vi "Hardware Device Get All Info.vi"(8 "error in":errorcluster, 9 "Terminals":tag[](array[tag]), 11 "NI PWM Output in":refnum<class "NI PWM Output.lvclass">) -> (0 "error out":errorcluster, 1 "CO.PhysicalChans":tag[](array[tag]), 3 "NI PWM Output out":refnum<class "NI PWM Output.lvclass">)   [LabVIEW 2023, in "HardwareAbstractionLayer_LVOOP.lvlib" / "NI PWM Output.lvclass"]
doc: "This VI Device Physical Channel Read"
uses:
  NI PWM Output.lvclass
  NI PWM Output.lvclass/NI PWM Output.ctl
  <resource>/objmgr/daqmx.rc
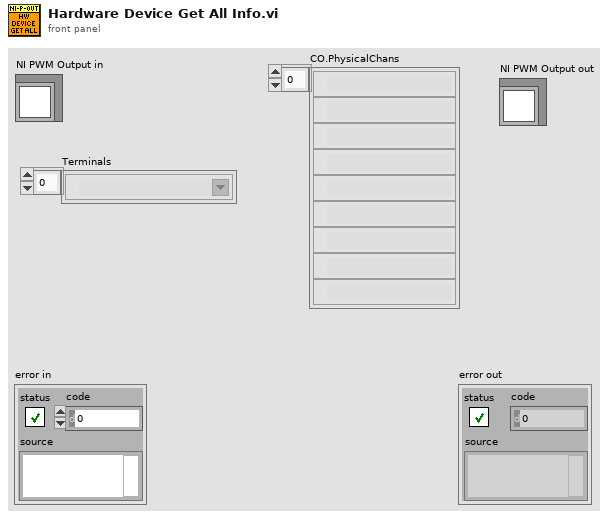
[diagram p1: front panel]
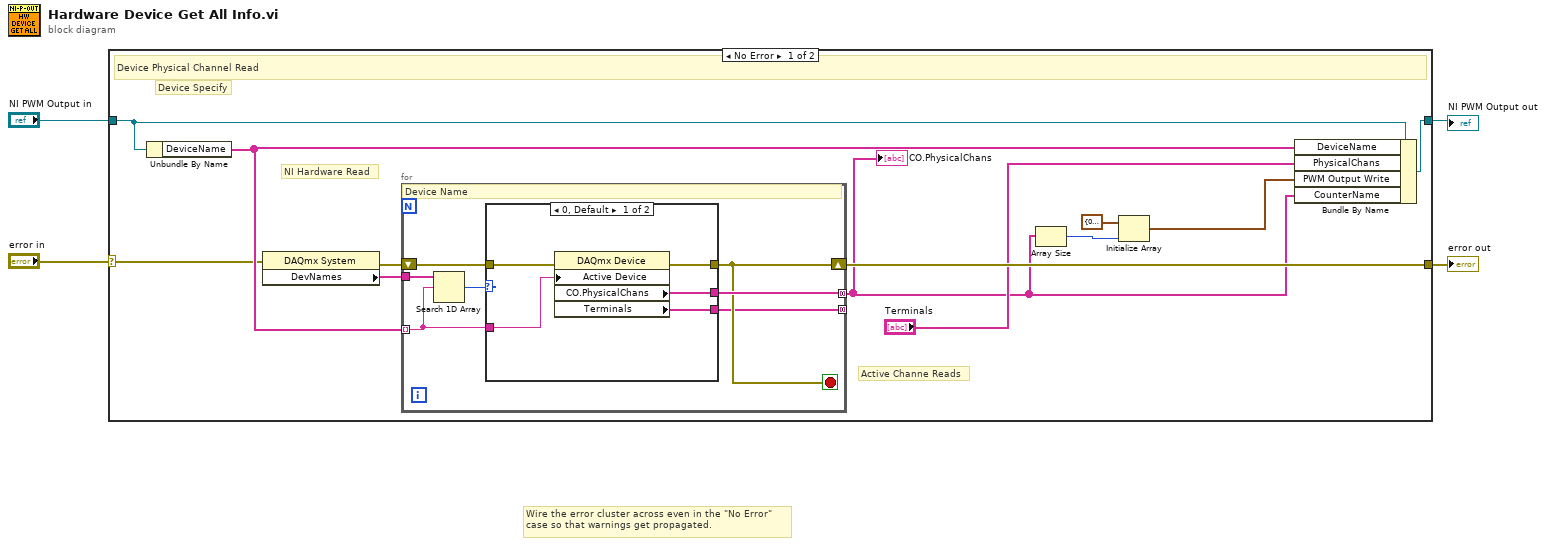
[diagram p0: block diagram]
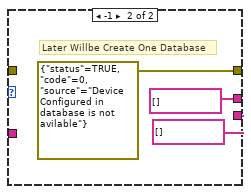
[diagram p2: hidden frame]
diagram:
  # "Wire the error cluster across even in the \"No Error\"\ncase so that warnings get propagated."
  n1 = case shown="No Error" "error in" {
    selector: "error in" -> [w7 w33]
    tunnel: [w8 w33] -> w3
    tunnel: [w13 w32] -> w1
    tunnel: "NI PWM Output in" -> [w12 w32]
    frame No Error {
      # "Active Channe Reads"
      # "Device Specify"
      # "NI Hardware Read"
      # "Device Physical Channel Read"
      n2 = Unbundle By Name(w12) -> ("DeviceName"=w16:tag[])
      n3 = property class="DAQmx System"(error in=w7) -> (error out=w14:errorcluster, "DevNames"=w15:tag[])  [unwired: 1 in, 1 out]
      n4 = for {
        tunnel: w16 -> [w20] mode=indexing
        tunnel: w15 -> [w21]
        tunnel: [w19] -> w5 mode=concatenating
        shift-right: [w18] -> w8
        shift-left: w14 -> [w22]
        tunnel: [w17] -> _ mode=concatenating
        stop <- w18 stop-if-true
        # "Device Name"
        n5 = Search 1D Array(1D array=w21, element=w20) -> (index of element=w23:i32)  [unwired: 1 in]
        n6 = case shown="0, Default" w23 {
          tunnel: w22 -> [w26 _]
          tunnel: [w25 errorcluster {"status"=TRUE, "code"=0, "source"="Device  Configured in database is not avilable"} ("error out")] -> w18
          tunnel: w20 -> [w28 _]
          tunnel: [w27 tag[] [] ("AI.PhysicalChans")] -> w19
          tunnel: [w24 tag[] [] ("Terminals")] -> w17
          frame 0, Default {
            n7 = property class="DAQmx Device"(error in=w26, "Active Device"=w28) -> (error out=w25:errorcluster, "CO.PhysicalChans"=w27:tag[], "Terminals"=w24:tag[])  [unwired: 1 in, 1 out]
          }
          frame -1 {
            # "Later Willbe Create One Database"
          }
        }
      }
      "CO.PhysicalChans" <- w5
      n8 = Array Size(array=w5) -> (size(s)=w11:i32)
      n9 = Initialize Array(cluster{"duty cycle":dbl, "frequency":dbl} {"duty cycle"=0.0, "frequency"=0.0} ("values"), w11) -> (w10:cluster{"duty cycle":dbl, "frequency":dbl}[])
      n10 = Bundle By Name(cluster=w12, "DeviceName"=w16, "PhysicalChans"="Terminals", "PWM Output Write"=w10, "CounterName"=w5) -> (w13:refnum<class "NI PWM Output.lvclass">)
    }
    frame Error {
    }
  }
  "error out" <- w3
  "NI PWM Output out" <- w1
